vi "SmartSyntax to FormatString.vi"(0 "Numeric Functions in":refnum<class "Numeric Functions.lvclass">, 5 "String":string, 11 "error in (no error)":errorcluster) -> (4 "Numeric Functions out":refnum<class "Numeric Functions.lvclass">, 6 "Scan Syntax Format":T1, 15 "error out":errorcluster)   [LabVIEW 2019, in "Numeric Functions.lvclass"]
uses:
  Numeric Functions.lvclass
  common/function utils/Scan Syntax Format.ctl
  functionsbase/functionbase.lvclass
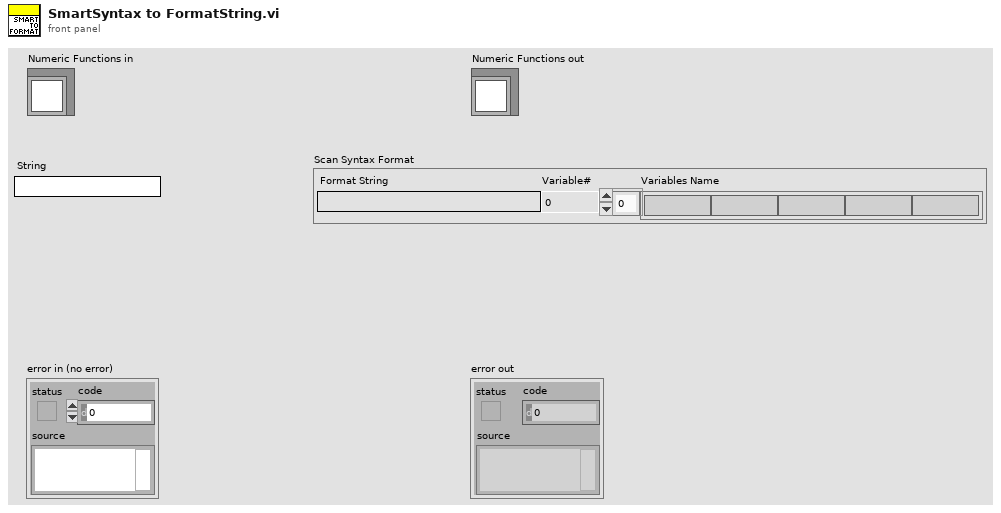
[diagram p1: front panel]
types:
  T1 = typedef "Scan Syntax Format.ctl" = cluster{"Format String":string, "Variable#":i32, "Variables Name":string[]}
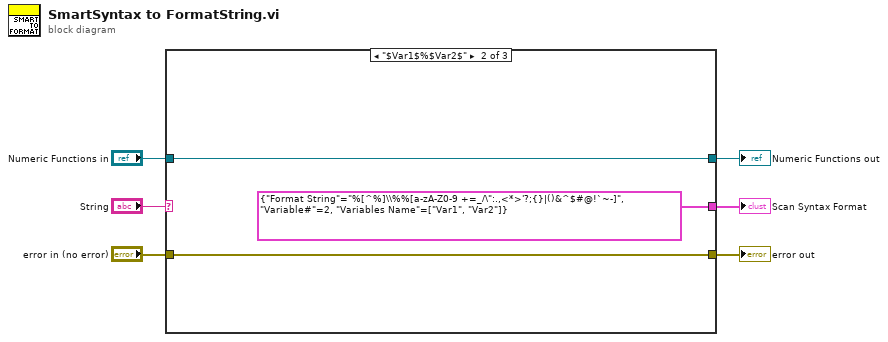
[diagram p0: block diagram]
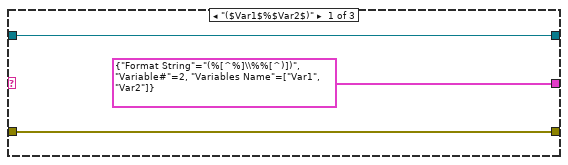
[diagram p2: hidden frame]
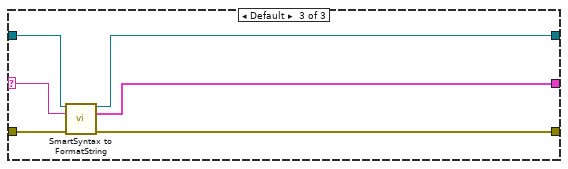
[diagram p3: hidden frame]
diagram:
  n1 = case shown="\"$Var1$%$Var2$\"" "String" {
    selector: "String" -> [_ _ w16]
    tunnel: "Numeric Functions in" -> [w9 w12 w18]
    tunnel: [w9 w12 w17] -> w5
    tunnel: [T1 {"Format String"="(%[^%]\\%%[^)])", "Variable#"=2, "Variables Name"=["Var1", "Var2"]} ("Scan Syntax Format") T1 {"Format String"="%[^%]\\%%[a-zA-Z0-9 +=_/\":.,<*>'?;{}|()&^$#@!`~-]", "Variable#"=2, "Variables Name"=["Var1", "Var2"]} ("Scan Syntax Format") w15] -> w3
    tunnel: "error in (no error)" -> [w8 w11 w14]
    tunnel: [w8 w11 w13] -> w1
    frame "($Var1$%$Var2$)" {
    }
    frame "$Var1$%$Var2$" {
    }
    frame Default {
      n2 = call-parent "SmartSyntax to FormatString.vi"("functionbase in"=w18, "String"=w16, "error in (no error)"=w14) -> ("functionbase out"=w17:refnum<class "Numeric Functions.lvclass">, "Scan Syntax Format"=w15:T1, "error out"=w13:errorcluster)  [unwired: 10 in]
    }
  }
  "error out" <- w1
  "Numeric Functions out" <- w5
  "Scan Syntax Format" <- w3
